vi "Create STRING.vi"(8 "error in (no error)":errorcluster, 10 "Descriptor":string, 11 "Value IN":dbl) -> (0 "error out":errorcluster, 3 "concatenated string":string)   [LabVIEW 2016]
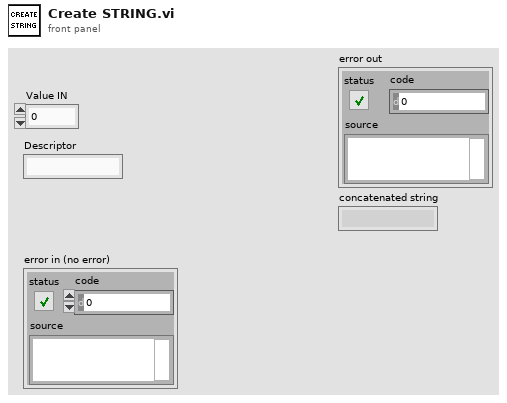
[diagram p1: front panel]
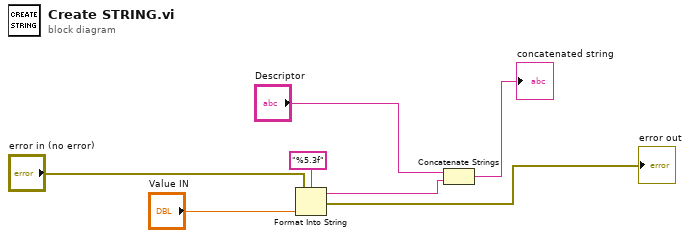
[diagram p0: block diagram]
diagram:
  n1 = Format Into String(format string="%5.3f", error in="error in (no error)", "Value IN") -> (resulting string=w5:string, error out=→"error out":errorcluster)  [unwired: 1 in]
  n2 = Concatenate Strings("Descriptor", w5) -> (→"concatenated string":string)
